vi "SubString.vi"(1 "Length":refnum<class "Abs_Numeric.lvclass">, 2 "Offset":refnum<class "Abs_Numeric.lvclass">, 3 "String":refnum<class "Abs_String.lvclass">) -> (0 "Result":refnum<class "Abs_String.lvclass">)   [LabVIEW 2021]
uses:
  Abs_Types/String/Abs_String.lvclass
  Abs_Types/Numeric/Abs_Numeric.lvclass
  Support/SubSet/Subset_STR.lvclass
  C:/Program Files (x86)/National Instruments/LabVIEW 2021/vi.lib/TSA/Abstract Data Classes/Abs_Types/String/Abs_String.lvclass
  Support/SubSet/Subset_STR.lvclass/Subset_STR.ctl
  Support/SubSet/Properties/Write String.vi
  Support/SubSet/Properties/Write Offset.vi
  Support/SubSet/Properties/Write Length.vi
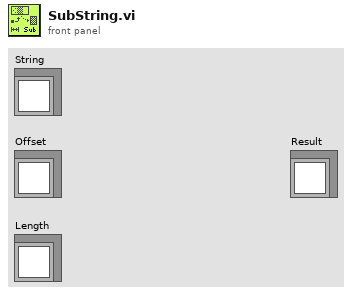
[diagram p1: front panel]
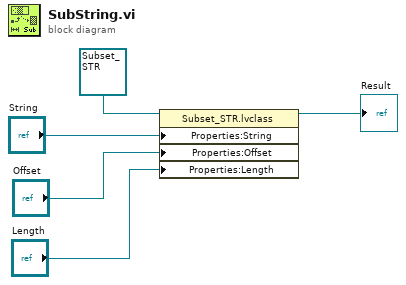
[diagram p0: block diagram]
diagram:
  n1 = property class="Subset_STR.lvclass"(reference=refnum<class "Subset_STR.lvclass"> refnum ("Subset_STR.lvclass"), "Properties:String"="String", "Properties:Offset"="Offset", "Properties:Length"="Length") -> (reference out=→"Result":refnum<class "Subset_STR.lvclass">)  [unwired: 1 in, 1 out]
